vi "Configurate_All_Main_v1.vi"(8 "error in":errorcluster, 9 "Time unit":string(combo)="ms", 10 "Config files paths":T1={"ZI config file (.ini)"="Config_Ver_1\\Zurich_params.ini", "Keithley config file (.ini)"="Config_Ver_1\\Keithley_params.ini", "Arduino config file (.ini)"="Config_Ver_1\\pulse_sequence.ini"}, 11 "Resources in":T6 {"ZI ModHandle"."ModHandle" format="0x%08x"; "ZI ModHandle"."Conn" format="0x%08x"; "ZI Handle"."Handle" format="0x%08x"; "ZI Handle"."Conn" format="0x%08x"}) -> (0 "error out":errorcluster, 1 "Init States":T4, 2 "Pulse sequence":T5[](array[typedef]) {"channel" min=2 max=13 step=1}, 3 "Resources out":T6 {"ZI ModHandle"."ModHandle" format="0x%08x"; "ZI ModHandle"."Conn" format="0x%08x"; "ZI Handle"."Handle" format="0x%08x"; "ZI Handle"."Conn" format="0x%08x"})   [LabVIEW 2021]
uses:
  Resources.ctl
  <instrlib>/Zurich Instruments LabOne/Public/ziTypeHandle.ctl
  <instrlib>/Zurich Instruments LabOne/Public/Modules/ziTypeModHandle.ctl
  Drivers/Arduino_Pulse_Generator/Configurate/Channel_Pulse_Stream.ctl
  Drivers/Arduino_Pulse_Generator/Configurate/Register_1.ctl
  Drivers/Arduino_Pulse_Generator/Configurate/Register_2.ctl
  Config_File_Paths.ctl
  <instrlib>/Zurich Instruments LabOne/Zurich Instruments LabOne.lvlib
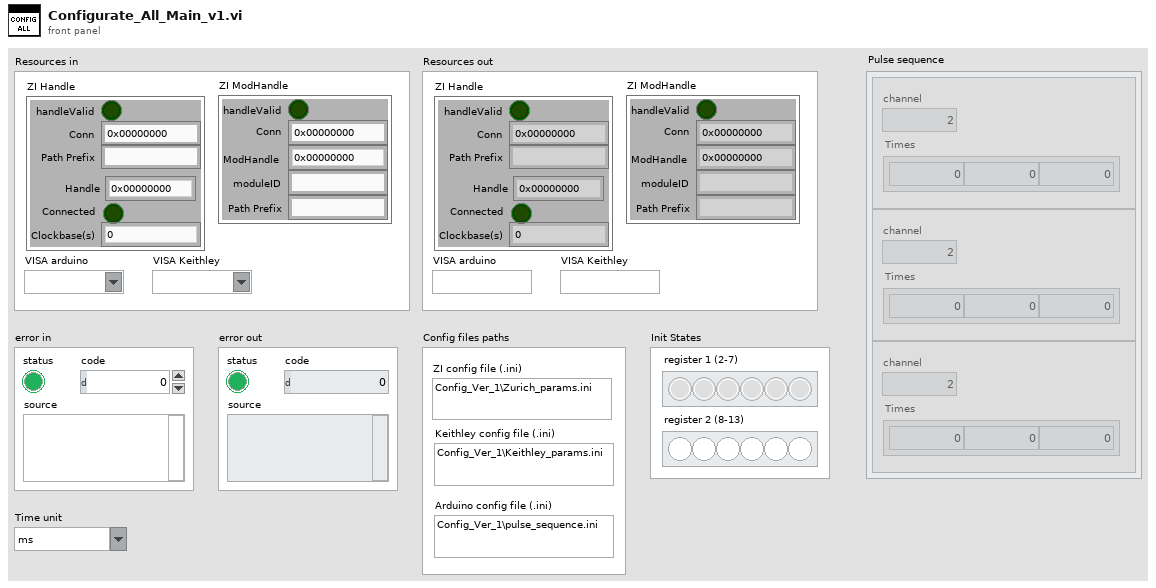
[diagram p1: front panel]
types:
  T1 = typedef "Config_File_Paths.ctl" = cluster{"ZI config file (.ini)":string, "Keithley config file (.ini)":string, "Arduino config file (.ini)":string}
  T2 = typedef "Register_1.ctl" = bool[]
  T3 = typedef "Register_2.ctl" = bool[]
  T4 = cluster{"register 1 (2-7)":T2, "register 2 (8-13)":T3}
  T5 = typedef "Channel_Pulse_Stream.ctl" = cluster{"Times":dbl[], "channel":u8}
  T6 = typedef "Resources.ctl" = cluster{"ZI Handle":T7, "ZI ModHandle":T8, "VISA arduino":refnum<visa-resource-name>, "VISA Keithley":refnum<visa-resource-name>}
  T7 = typedef "Zurich Instruments LabOne.lvlib/ziTypeHandle.ctl" = cluster{"handleValid":bool, "Conn":u64, "Path Prefix":string, "Handle":u64, "Connected":bool, "Clockbase(s)":dbl}
  T8 = typedef "Zurich Instruments LabOne.lvlib/ziTypeModHandle.ctl" = cluster{"handleValid":bool, "Conn":u64, "ModHandle":u64, "moduleID":string, "Path Prefix":string}
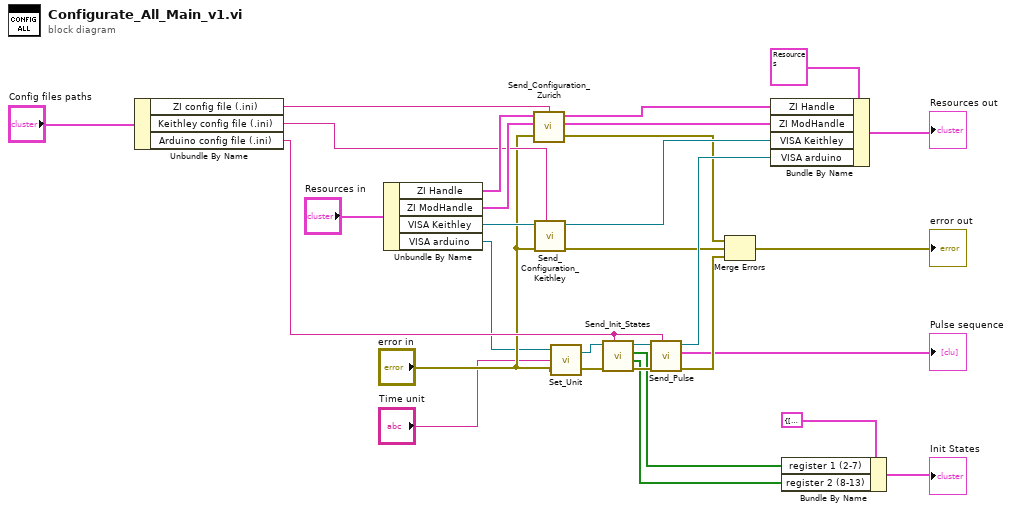
[diagram p0: block diagram]
diagram:
  n1 = Unbundle By Name("Config files paths") -> ("ZI config file (.ini)"=w14:string, "Keithley config file (.ini)"=w13:string, "Arduino config file (.ini)"=w12:string)
  n2 = Unbundle By Name("Resources in") -> ("ZI Handle"=w26:T7, "ZI ModHandle"=w25:T8, "VISA Keithley"=w27:refnum<visa-resource-name>, "VISA arduino"=w7:refnum<visa-resource-name>)
  n3 = call "Send_Configuration_Zurich.vi"("Filename (.ini)"=w14, "Handle In"=w26, "ModHandle In"=w25, "error in"="error in") -> ("Handle Out"=w19:T7, "ModHandle Out"=w20:T8, "error out"=w16:errorcluster)  [unwired: 1 in]
  n4 = call "Send_Configuration_Keithley.vi"("Filename (.ini)"=w13, "error in"="error in", "Keithley VISA in"=w27) -> ("error out"=w17:errorcluster, "Keithley VISA out"=w21:refnum<visa-resource-name>)  [unwired: 4 in, 3 out]
  n5 = call "Set_Unit.vi"("error in"="error in", "Unit"="Time unit", "VISA arduino in"=w7) -> ("error out"=w9:errorcluster, "VISA arduino out"=w10:refnum<visa-resource-name>)
  n6 = call "Send_Init_States.vi"("Filename (.ini)"=w12, "error in"=w9, "VISA arduino in"=w10) -> ("error out"=w29:errorcluster, "register 2 (8-13)"=w4:T3, "register 1 (2-7)"=w3:T2, "VISA arduino out"=w30:refnum<visa-resource-name>)  [unwired: 5 in]
  n7 = call "Send_Pulse.vi"("Filename (.ini)"=w12, "error in"=w29, "VISA arduino in"=w30) -> ("error out"=w18:errorcluster, "Pulse sequence"=→"Pulse sequence":T5[], "VISA arduino out"=w22:refnum<visa-resource-name>)  [unwired: 6 in]
  n8 = Merge Errors(w16, w17, w18) -> (→"error out":errorcluster)
  n9 = Bundle By Name(cluster=T6 {"ZI Handle"={"handleValid"=FALSE, "Conn"=0, "Path Prefix"="", "Handle"=0, "Connected"=FALSE, "Clockbase(s)"=0.0}, "ZI ModHandle"={"handleValid"=FALSE, "Conn"=0, "ModHandle"=0, "moduleID"="", "Path Prefix"=""}, "VISA arduino"="", "VISA Keithley"=""} ("Resources"), "ZI Handle"=w19, "ZI ModHandle"=w20, "VISA Keithley"=w21, "VISA arduino"=w22) -> (→"Resources out":T6)
  n10 = Bundle By Name(cluster=T4 {"register 1 (2-7)"=[], "register 2 (8-13)"=[FALSE, FALSE, FALSE, FALSE, FALSE, FALSE]} ("Init States"), "register 1 (2-7)"=w3, "register 2 (8-13)"=w4) -> (→"Init States":T4)
